vi "StopModByModuleID.vi"(8 "ErrorArray In":errorcluster[](array[cluster]), 10 "Module ID":i32=-1, 11 "Test.lvclass":refnum<class "Test.lvclass">) -> (0 "ErrorArray Out":errorcluster[](array[cluster]), 3 "Test.lvclass":refnum<class "Test.lvclass">)   [LabVIEW 2018, in "Test.lvclass"]
doc: "Stops all modules based on the Test Class information (Clone Registration, Module ID, and Module list)."
uses:
  Test.lvclass
  Test.lvclass/Test.ctl
  Accessors/Write CloneReg.vi
  Accessors/Write ModuleIDs.vi
  Accessors/Write ModuleList.vi
  Accessors/Read CloneReg.vi
  Accessors/Read ModuleIDs.vi
  Accessors/Read ModuleList.vi
  <userlib>/NIST/ModuleAdminLib/CloneRegistration/CloneRegistration.lvclass
  <userlib>/NIST/NISTErrorLib/NISTErrorLib.lvlib
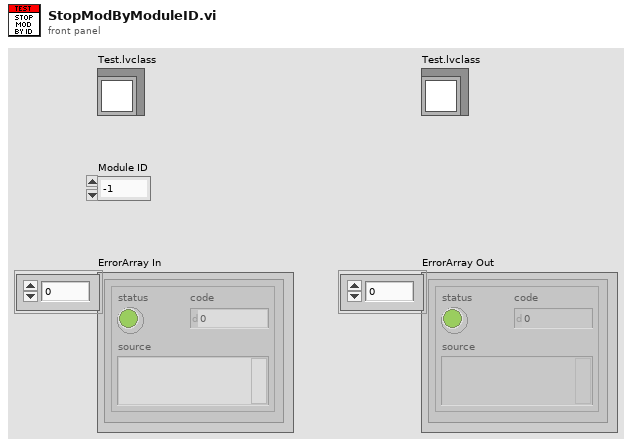
[diagram p1: front panel]
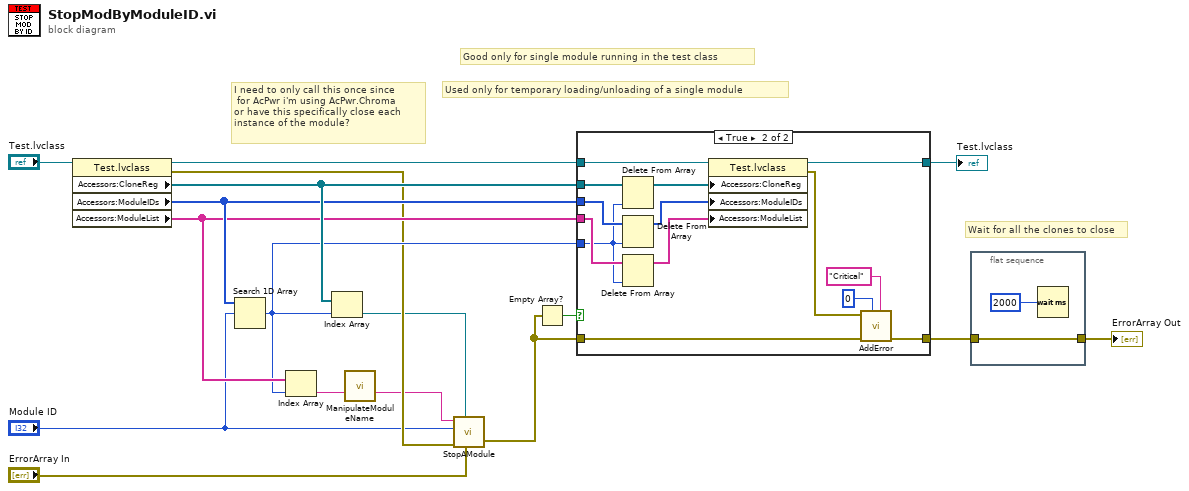
[diagram p0: block diagram]
diagram:
  # "Used only for temporary loading/unloading of a single module"
  # "Good only for single module running in the test class"
  # "I need to only call this once since\n for AcPwr i'm using AcPwr.Chroma\nor have this specifically close each \ninstance of the module?"
  # "Wait for all the clones to close"
  n1 = property class="Test.lvclass"(reference="Test.lvclass") -> (reference out=w14:refnum<class "Test.lvclass">, error out=w5:errorcluster, "Accessors:CloneReg"=w12:refnum<data-value>[], "Accessors:ModuleIDs"=w11:i32[], "Accessors:ModuleList"=w10:string[])  [unwired: 1 in]
  n2 = Search 1D Array(1D array=w11, element="Module ID") -> (index of element=w8:i32)  [unwired: 1 in]
  n3 = Index Array(array=w10, index=w8) -> (element=w15:string)
  n4 = Index Array(array=w12, index=w8) -> (element=w2:refnum<data-value>)
  n5 = call "ManipulateModuleName.vi"("ModuleListSingleEntry"=w15) -> ("BeforeMatch:ModuleListSingleEntry"=w1:string)  [unwired: 9 in, 5 out]
  n6 = call "StopAModule.vi"("ErrorArray In"="ErrorArray In", "Module Clone Reg"=w2, "error in (no error)"=w5, "Module ID"="Module ID", "Module Name (e.g. Sensor, Digitizer, etc.)"=w1) -> ("ErrorArray Out"=w7:errorcluster[])  [unwired: 6 in]
  n7 = Empty Array?(array=w7) -> (empty?=w13:bool)
  n8 = case shown="True" w13 {
    tunnel: w14 -> [w19 w33]
    tunnel: w12 -> [_ w31]
    tunnel: w11 -> [_ w30]
    tunnel: w10 -> [_ w29]
    tunnel: [w19 w32] -> w9
    tunnel: w8 -> [_ w28]
    tunnel: w7 -> [w18 w21]
    tunnel: [w18 w20] -> w6
    frame False {
    }
    frame True {
      n9 = Delete From Array(array=w31, index=w28) -> (array with subset deleted=w27:refnum<data-value>[])  [unwired: 1 in, 1 out]
      n10 = Delete From Array(array=w30, index=w28) -> (array with subset deleted=w26:i32[])  [unwired: 1 in, 1 out]
      n11 = Delete From Array(array=w29, index=w28) -> (array with subset deleted=w25:string[])  [unwired: 1 in, 1 out]
      n12 = property class="Test.lvclass"(reference=w33, "Accessors:CloneReg"=w27, "Accessors:ModuleIDs"=w26, "Accessors:ModuleList"=w25) -> (reference out=w32:refnum<class "Test.lvclass">, error out=w22:errorcluster)  [unwired: 1 in]
      n13 = call <userlib>:"AddError.vi"("Severity"="Critical", "Priority"=u8 0, "ErrorArray In"=w21, "error in (no error)"=w22) -> ("ErrorArray Out"=w20:errorcluster[])  [unwired: 6 in, 1 out]
    }
  }
  "Test.lvclass" <- w9
  n14 = flat-sequence {
    tunnel: [w35] -> w16
    tunnel: w6 -> [w35]
    frame #0 {
      n15 = Wait (ms)(milliseconds to wait=u32 2000) -> ()  [unwired: 1 out]
    }
  }
  "ErrorArray Out" <- w16
